vi "save chromatogram.vi"(6 "GC record":T1 {"delta x" format="%.2f"; "chromatogram 1" format="%.2f"}) -> (2 "GC record":T1 {"delta x" format="%.2f"; "chromatogram 1" format="%.2f"})   [LabVIEW 2012]
uses:
  GC record.ctl
panel:
  in  "CANCELED":bool
  in  "CANCEL":bool
  in  "?":bool
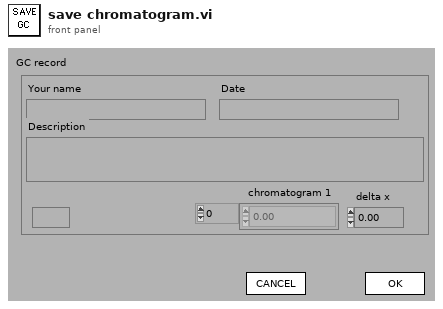
[diagram p1: front panel]
types:
  T1 = typedef "GC record.ctl" = cluster{"chromatogram 1":dbl[], "Your name":string, "Description":string, "Date":string, "delta x":dbl, "Det in use":string}
  T2 = enum16{"open", "open or create", "create or replace", "create", "open (read only)"}
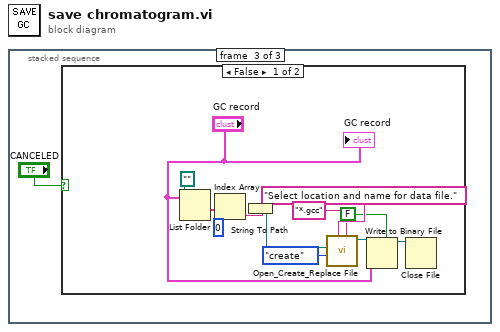
[diagram p0: block diagram]
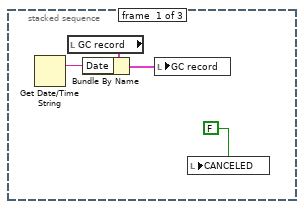
[diagram p2: hidden frame]
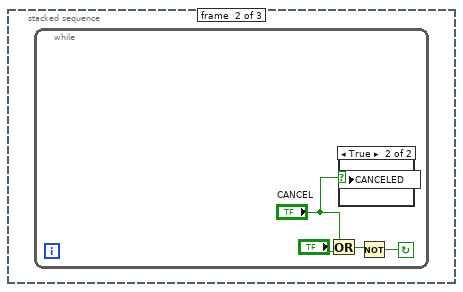
[diagram p3: hidden frame]
diagram:
  n1 = stacked-sequence {
    frame #0 {
      n2 = Get Date/Time String() -> (date string=w2:string)  [unwired: 3 in, 1 out]
      n3 = local read "GC record"() -> (w4:T1)
      n4 = Bundle By Name(cluster=w4, "Date"=w2) -> (w3:T1)
      n5 = local write "GC record"(w3) -> ()
      n6 = local write "CANCELED"(FALSE) -> ()
    }
    frame #1 {
      n7 = while {
        stop <- w7 continue-if-true
        n8 = Or(x="CANCEL", y="?") -> (x .or. y?=w6:bool)
        n9 = case shown="True" "CANCEL" {
          selector: "CANCEL" -> [_ w9]
          frame False {
          }
          frame True {
            n10 = local write "CANCELED"(w9) -> ()
          }
        }
        n11 = Not(x=w6) -> (.not. x?=w7:bool)
      }
    }
    frame #2 {
      n12 = case shown="False" "CANCELED" {
        frame False {
          n13 = List Folder(datalog type="GC record", path=path "") -> (folder names=w19:string[])  [unwired: 2 in, 3 out]
          n14 = Index Array(array=w19, index=0) -> (element=w21:string)
          n15 = String To Path(string=w21) -> (path=w13:path)
          n16 = call <vilib>:"Open_Create_Replace File.vi"("pattern"="*.gcc", "prompt"="Select location and name for data file.", "function (open:0)"=T2."create", "start path  (Not A Path)"=w13) -> ("refnum"=w16:refnum<file>)  [unwired: 4 in, 3 out]
          n17 = Write to Binary File(file (use dialog)=w16, data="GC record", 5:FALSE ("prepend array or string size? (T)")) -> (refnum out=w18:refnum<file>)  [unwired: 3 in, 2 out]
          n18 = Close File(refnum=w18) -> ()  [unwired: 1 in, 2 out]
          "GC record" <- "GC record"
        }
        frame True {
        }
      }
    }
  }
